vi "Get Class Name.vi"(8 "error in (no error)":errorcluster, 11 "Abs_Type in":refnum<class "Abs_Type.lvclass">) -> (0 "error out":errorcluster, 3 "class name":string)   [LabVIEW 2021, in "Abs_Type.lvclass"]
uses:
  Abs_Type.lvclass
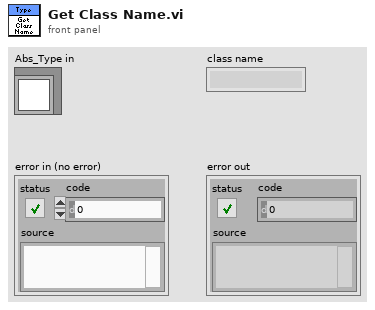
[diagram p1: front panel]
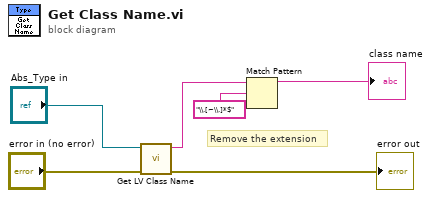
[diagram p0: block diagram]
diagram:
  # "Remove the extension"
  n1 = call <vilib>:"Get LV Class Name.vi"("error in (no error)"="error in (no error)", "object"="Abs_Type in") -> ("error out"=→"error out":errorcluster, "class name"=w5:string)  [unwired: 8 in]
  n2 = Match Pattern(string=w5, regular expression="\\.[~\\.]*$") -> (before substring=→"class name":string)  [unwired: 4 out]
